vi "LabView_Pulsed_Single_LED.vi"() -> ()   [LabVIEW 2020]
uses:
  <vilib>/Instr/_visa.llb/VISA Configure Serial Port (Instr).vi
  <vilib>/measure/NI_MABase.lvlib
panel:
  in  "sampling info":cluster{"Fs":dbl, "#s":dbl}={"Fs"=1000.0, "#s"=1000.0} {"Fs" format="%.2p"}
  out "Waveform Chart":waveform(dbl)(graph)
  in  "signal type":T1(ring)
  out "Boolean":bool
  in  "Frequency":dbl=10.0 min=0.0 max=3000.0 step=1.0
  in  "VISA resource name":refnum<visa-resource-name>
  in  "stop":bool
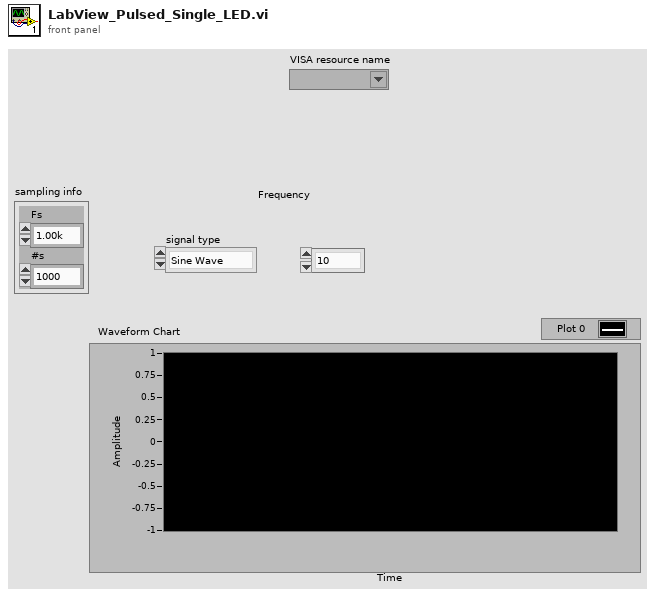
[diagram p1: front panel]
types:
  T1 = enum16{"Sine Wave", "Triangle Wave", "Square Wave", "Sawtooth Wave"}
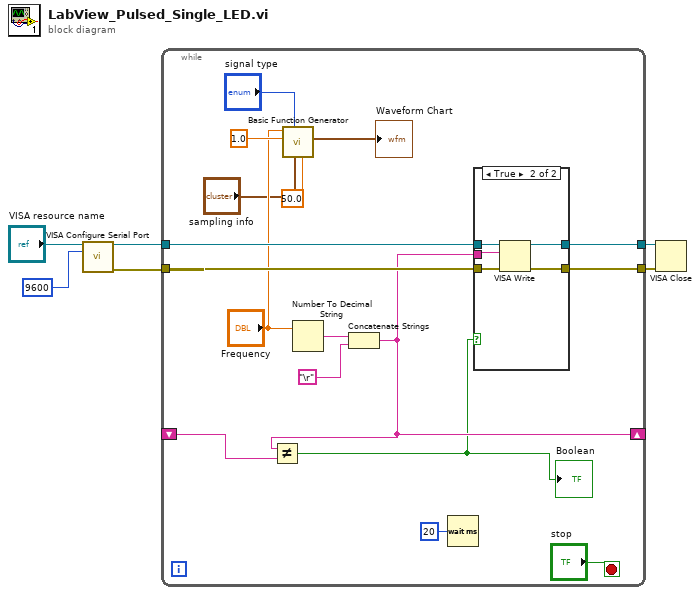
[diagram p0: block diagram]
diagram:
  n1 = call-poly "VISA Configure Serial Port"("VISA resource name"="VISA resource name", "baud rate (9600)"=u32 9600) -> ("VISA resource name out"=w2:refnum<visa-resource-name>, "error out"=w1:errorcluster)  [unwired: 12 in]
  n2 = while {
    tunnel: w2 -> [w20]
    tunnel: [w19] -> w5
    tunnel: w1 -> [w18]
    tunnel: [w17] -> w4
    shift-right: [w14] -> _
    shift-left: _ -> [w15]
    stop <- "stop" stop-if-true
    n3 = call <vilib>:"Basic Function Generator.vi"("square wave duty cycle (%)"=50.0, "sampling info"="sampling info", "signal type"="signal type", "amplitude"=1.0, "frequency"="Frequency") -> ("signal out"=→"Waveform Chart":waveform(dbl))  [unwired: 4 in, 2 out]
    n4 = Number To Decimal String(number="Frequency") -> (decimal integer string=w22:string)  [unwired: 1 in]
    n5 = Concatenate Strings(w22, "\r") -> (w14:string)
    n6 = Not Equal?(x=w14, y=w15) -> (x != y?=w13:bool)
    "Boolean" <- w13
    n7 = Wait (ms)(milliseconds to wait=u32 20) -> ()  [unwired: 1 out]
    n8 = case shown="True" w13 {
      tunnel: w20 -> [w25 w30]
      tunnel: [w25 w29] -> w19
      tunnel: w18 -> [w24 w28]
      tunnel: [w24 w27] -> w17
      tunnel: w14 -> [_ w26]
      frame False {
      }
      frame True {
        n9 = VISA Write(VISA resource name=w30, write buffer=w26, error in (no error)=w28) -> (VISA resource name out=w29:refnum<visa-resource-name>, error out=w27:errorcluster)  [unwired: 1 out]
      }
    }
  }
  n10 = VISA Close(VISA resource name=w5, error in (no error)=w4) -> ()  [unwired: 1 out]
